vi "example_get_device_digital_output_values.vi"() -> ()   [LabVIEW 2012]
doc: "EXAMPLE: Get Device Digital Outputs\n\nThis example VI demonstrates how to retrieve the current status value(s) of the device's digital output channels. \n\nProduced By:\n\nChristopher Lemieux\nKod Integrations, LLC\n4835 Marianne Drive\nMount Airy, MD 21771\nhttp://www.kodintegrations.com\nemail: clemieux@kodintegrations.com\nphone: (240) 687-1288"
uses:
  support/controls/digital_output_item_group.ctl
  support/controls/digital_output_items.ctl
panel:
  in  "get_all? (def=F)":bool
  in  "do (single)":T1
  out "dig_out_val (single only)":bool
  out "do_items":T2[](array[typedef])
  in  "device_index (def=0)":i32
  out "error out":errorcluster
  in  "error in (no error)":errorcluster
  # "If just retrieving (1) DO value, select the value you wish to retrieve\nthen RUN the VI"
  # "FALSE"
  # "If retrieving ALL items\nsimply RUN the VI..."
  # "TRUE"
  # "FIRST determine if you want\nto retrieve just (1) digital\noutput value, or all of them.\n\nget ALL = TRUE\nget ONE = FALSE"
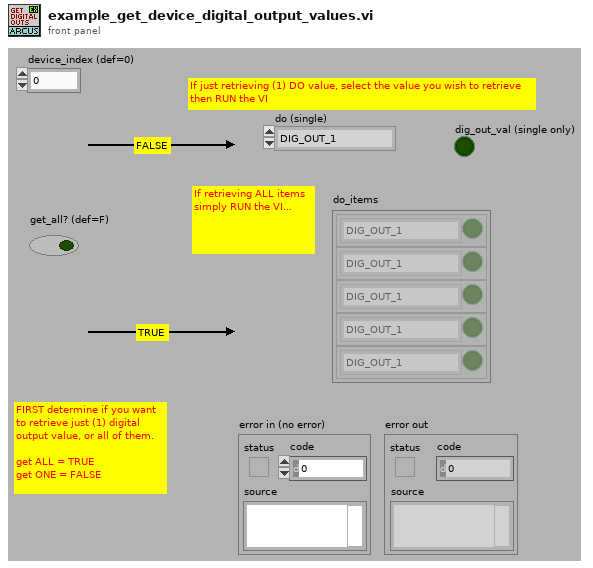
[diagram p1: front panel]
types:
  T1 = typedef "digital_output_items.ctl" = enum16{"DIG_OUT_1", "DIG_OUT_2"}
  T2 = typedef "digital_output_item_group.ctl" = cluster{"item":T1, "status":bool}
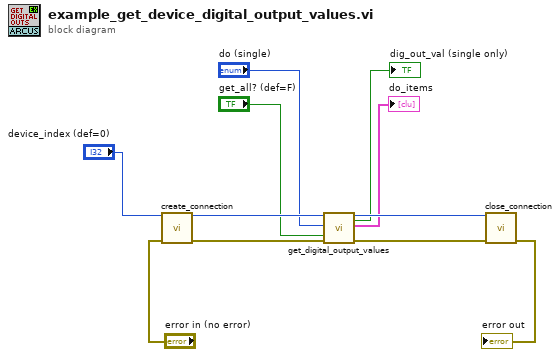
[diagram p0: block diagram]
diagram:
  n1 = call "create_connection.vi"("device_index (def=0)"="device_index (def=0)", "error in (no error)"="error in (no error)") -> ("reference"=w7:i32, "error out"=w8:errorcluster)  [unwired: 12 in]
  n2 = call "get_digital_output_values.vi"("reference (in)"=w7, "do (single)"="do (single)", "get_all? (def=F)"="get_all? (def=F)", "error in (no error)"=w8) -> ("reference (dup)"=w6:i32, "dig_out_val (single only)"=→"dig_out_val (single only)":bool, "do_items"=→"do_items":T2[], "error out"=w5:errorcluster)  [unwired: 11 in, 1 out]
  n3 = call "close_connection.vi"("reference"=w6, "error in (no error)"=w5) -> ("error out"=→"error out":errorcluster)  [unwired: 13 in]
